vi "Set Timer Period.vi"(6 "Name":string, 7 "Metadata":string, 8 "error in (no error)":errorcluster, 11 "Period [s]":dbl=nan format="%#_13g") -> (0 "error out":errorcluster)   [LabVIEW 2015, in "Task Scheduler Actor API.lvclass"]
uses:
  Task Scheduler Actor API.lvclass
  Actor/Timer Config.ctl
  Re-use Libraries/Minimal Actor Framework/Messaging/Message/Message.lvclass/Message.ctl
  Globals.vi
  Re-use Libraries/Minimal Actor Framework/Messaging/Message/Message.lvclass
  Actor/Task Scheduler Actor.lvclass
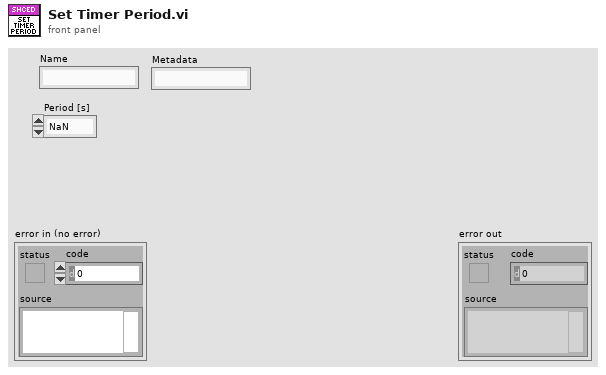
[diagram p1: front panel]
types:
  T1 = typedef "Task Scheduler Actor.lvclass/Timer Config.ctl" = cluster{"Name":string, "Period [s]":dbl, "Enabled":bool, "Metadata":string}
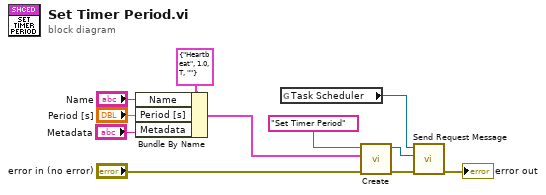
[diagram p0: block diagram]
diagram:
  n1 = Bundle By Name(cluster=T1 {"Name"="Heartbeat", "Period [s]"=1.0, "Enabled"=TRUE, "Metadata"=""} ("Timer Config"), "Name"="Name", "Period [s]"="Period [s]", "Metadata"="Metadata") -> (w4:T1)
  n2 = global read "Globals.vi" "Task Scheduler"() -> (w6:refnum<class "Task Scheduler Actor API.lvclass">)
  n3 = call "Create.vi"("error in (no error)"="error in (no error)", "Data"=w4, "Name"="Set Timer Period" ("Parameter")) -> ("error out"=w7:errorcluster, "Message out"=w8:refnum<class "Message.lvclass">)  [unwired: 7 in]
  n4 = call-dynamic "Send Request Message.vi"("error in (no error)"=w7, "Message"=w8, "Actor API in"=w6) -> ("error out"=→"error out":errorcluster)  [unwired: 8 in]
